vi "Read Userinfo.vi"(8 "error in (no error)":errorcluster, 11 "[Data] Userinfo Binary in":refnum<class "[Data] Userinfo Binary.lvclass">) -> (0 "error out":errorcluster, 3 "[Data] Userinfo Binary out":refnum<class "[Data] Userinfo Binary.lvclass">)   [LabVIEW 2020, in "[Data] Userinfo Binary.lvclass"]
uses:
  [Data] Userinfo Binary.lvclass
  [Data] Userinfo Binary.lvclass/[Data] Userinfo Binary.ctl
  <vilib>/YU/YU-Encrypt/AES/AES.lvclass
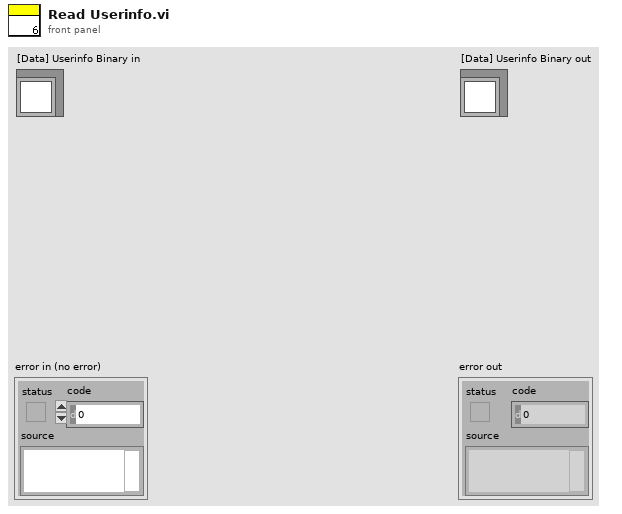
[diagram p1: front panel]
types:
  T1 = enum16{"open", "replace", "create", "open or create", "replace or create", "replace or create with confirmation"}
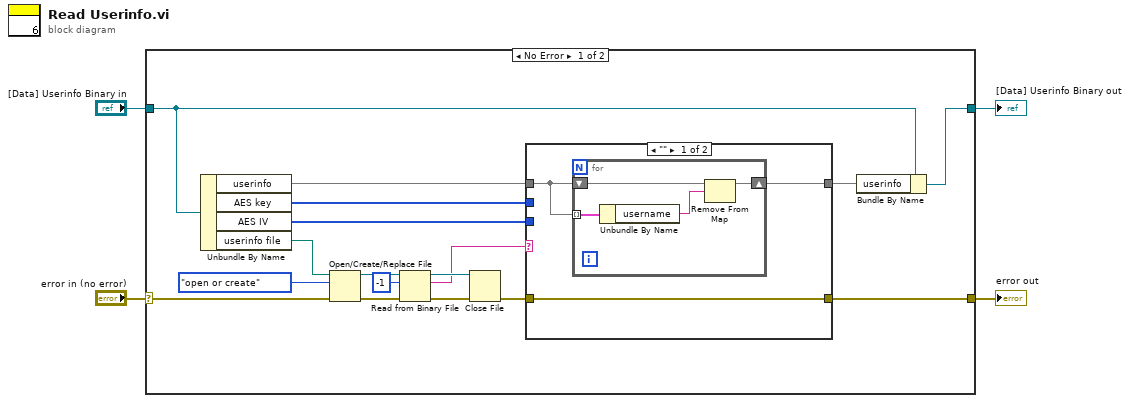
[diagram p0: block diagram]
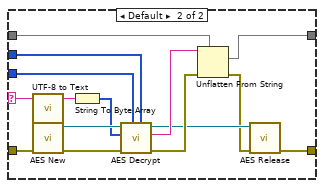
[diagram p2: hidden frame]
diagram:
  n1 = case shown="No Error" "error in (no error)" {
    selector: "error in (no error)" -> [w21 w45]
    tunnel: [w8 w45] -> w3
    tunnel: [w5 w44] -> w1
    tunnel: "[Data] Userinfo Binary in" -> [w7 w44]
    frame No Error {
      n2 = Unbundle By Name(w7) -> ("userinfo"=w9:map{string, cluster{"password":string}}, "AES key"=w10:u8[], "AES IV"=w11:u8[], "userinfo file"=w20:path)
      n3 = Open/Create/Replace File(file path (use dialog)=w20, error in=w21, operation (0:open)=T1."open or create") -> (refnum out=w17:refnum<file>, error out=w18:errorcluster)  [unwired: 3 in, 1 out]
      n4 = Read from Binary File(8:w18, 10:-1 ("count (1)"), 11:w17) -> (0:w15:errorcluster, 2:w12:string, 3:w14:refnum<file>)  [unwired: 3 in, 1 out]
      n5 = Close File(refnum=w14, error in=w15) -> (error out=w13:errorcluster)  [unwired: 1 out]
      n6 = case shown="\"\"" w12 {
        selector: w12 -> [_ w39]
        tunnel: w13 -> [w24 w38]
        tunnel: [w24 w30] -> w8
        tunnel: w11 -> [_ w40]
        tunnel: w10 -> [_ w41]
        tunnel: w9 -> [w23 w35]
        tunnel: [w22 w29] -> w6
        frame "" {
          n7 = for {
            shift-right: [w25] -> w22
            shift-left: w23 -> [w27]
            tunnel: w23 -> [w28] mode=indexing
            n8 = Unbundle By Name(w28) -> ("username"=w26:string)
            n9 = Remove From Map(10:w26, 11:w27) -> (3:w25:map{string, cluster{"password":string}})  [unwired: 2 out]
          }
        }
        frame Default {
          n10 = call <vilib>:"UTF-8 to Text.vi"("utf-8 text"=w39) -> ("text"=w37:string)  [unwired: 4 in]
          n11 = call <vilib>:"AES New.vi"("error in (no error)"=w38) -> ("error out"=w43:errorcluster, "AES out"=w42:refnum<class "AES.lvclass">)  [unwired: 9 in]
          n12 = String To Byte Array(string=w37) -> (unsigned byte array=w36:u8[])
          n13 = call <vilib>:"AES Decrypt.vi"("Key"=w41, "IV"=w40, "error in (no error)"=w43, "encrypted data"=w36, "AES in"=w42) -> ("error out"=w33:errorcluster, "data"=w34:string, "AES out"=w32:refnum<class "AES.lvclass">)  [unwired: 4 in]
          n14 = Unflatten From String(type=w35, binary string=w34, error in (no error)=w33) -> (value=w29:map{string, cluster{"password":string}}, error out=w31:errorcluster)  [unwired: 2 in, 1 out]
          n15 = call <vilib>:"AES Release.vi"("error in (no error)"=w31, "AES in"=w32) -> ("error out"=w30:errorcluster)  [unwired: 9 in]
        }
      }
      n16 = Bundle By Name(cluster=w7, "userinfo"=w6) -> (w5:refnum<class "[Data] Userinfo Binary.lvclass">)
    }
    frame Error {
    }
  }
  "error out" <- w3
  "[Data] Userinfo Binary out" <- w1
